vi "get Position (As Cluster).vi"(11 "Element in":refnum<class "Element.lvclass">) -> (3 "Position":T1)   [LabVIEW 2021, in "Element.lvclass"]
uses:
  Element.lvclass
  Element.lvclass/Element.ctl
  Motion/Motion.lvclass/Motion.ctl
  Vector 2D/Vector 2D.lvclass/Vector 2D.ctl
  Motion/Motion.lvclass
  Vector 2D/Vector 2D.lvclass
  LabSDL2/Source/Libraries/SDL2 Utility/Point (I32).ctl
  LabSDL2/Source/Libraries/SDL2 Utility/SDL2 Utility.lvlib
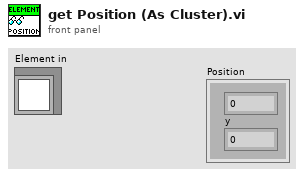
[diagram p1: front panel]
types:
  T1 = typedef "SDL2 Utility.lvlib/Point (I32).ctl" = cluster{"x":i32, "y":i32}
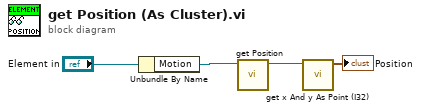
[diagram p0: block diagram]
diagram:
  n1 = Unbundle By Name("Element in") -> ("Motion"=w3:refnum<class "Motion.lvclass">)
  n2 = call "get Position.vi"("Motion in"=w3) -> ("Displacement"=w2:refnum<class "Vector 2D.lvclass">)  [unwired: 10 in]
  n3 = call "get x And y As Point (I32).vi"("Vector 2D in"=w2) -> ("Point"=→"Position":T1)  [unwired: 10 in]
